vi "SELECTOR.vi"(9 "Orden":T2(array[ring])=[enum."espejos", enum."voltaje", enum."polarizador", enum."potenciometro y lockin"], 10 "arreglo opciones":bool[](array[boolean])=[FALSE, FALSE, TRUE, FALSE, TRUE]) -> (2 "Enum":T1(ring))   [LabVIEW 2016]
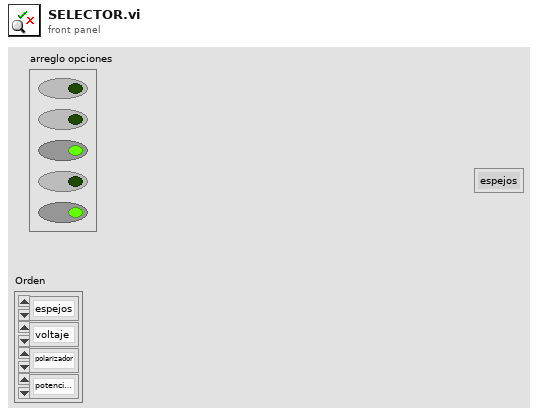
[diagram p1: front panel]
types:
  T1 = enum16{"espejos", "polarizador", "voltaje", "potenciometro y lockin", "CCD"}
  T2 = enum16{"espejos", "polarizador", "voltaje", "potenciometro y lockin", "CCD"}[]
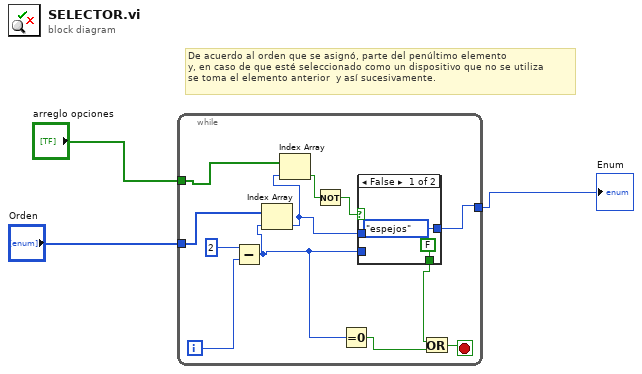
[diagram p0: block diagram]
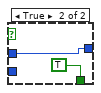
[diagram p2: hidden frame]
diagram:
  # "De acuerdo al orden que se asignó, parte del penúltimo elemento\ny, en caso de que esté seleccionado como un dispositivo que no se utiliza\nse toma el elemento anterior  y así sucesivamente."
  n1 = while {
    tunnel: "Orden" -> [w5]
    tunnel: "arreglo opciones" -> [w15]
    tunnel: [w12] -> w1
    i -> [w13]
    stop <- w11 stop-if-true
    n2 = Subtract(x=2, y=w13) -> (x-y=w6:i32)
    n3 = Index Array(array=w5, index=w6) -> (element=w4:T1)
    n4 = Index Array(array=w15, index=w4) -> (element=w8:bool)
    n5 = Not(x=w8) -> (.not. x?=w7:bool)
    n6 = Equal To 0?(x=w6) -> (x = 0?=w9:bool)
    n7 = case shown="False" w7 {
      tunnel: w6 -> [_ _]
      tunnel: [T1."espejos" ("Enum") w18] -> w12
      tunnel: [FALSE TRUE] -> w10
      tunnel: w4 -> [_ w18]
      frame False {
      }
      frame True {
      }
    }
    n8 = Or(x=w10, y=w9) -> (x .or. y?=w11:bool)
  }
  "Enum" <- w1
